vi "Move Beam.vi"(10 "Beam":refnum<class "Beam.lvclass">, 11 "Maze In":refnum<class "Maze.lvclass">) -> (2 "Beams":refnum<class "Beam.lvclass">[](array[class]), 3 "Maze Out":refnum<class "Maze.lvclass">)   [LabVIEW 2021, in "Maze.lvclass"]
uses:
  Maze.lvclass
  Beam/Beam.lvclass
  Maze.lvclass/Maze.ctl
  Beam/Beam.lvclass/Beam.ctl
  Beam/Read Row.vi
  Beam/Read Col.vi
  Beam/Read Direction.vi
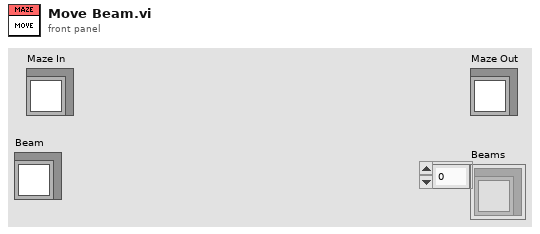
[diagram p1: front panel]
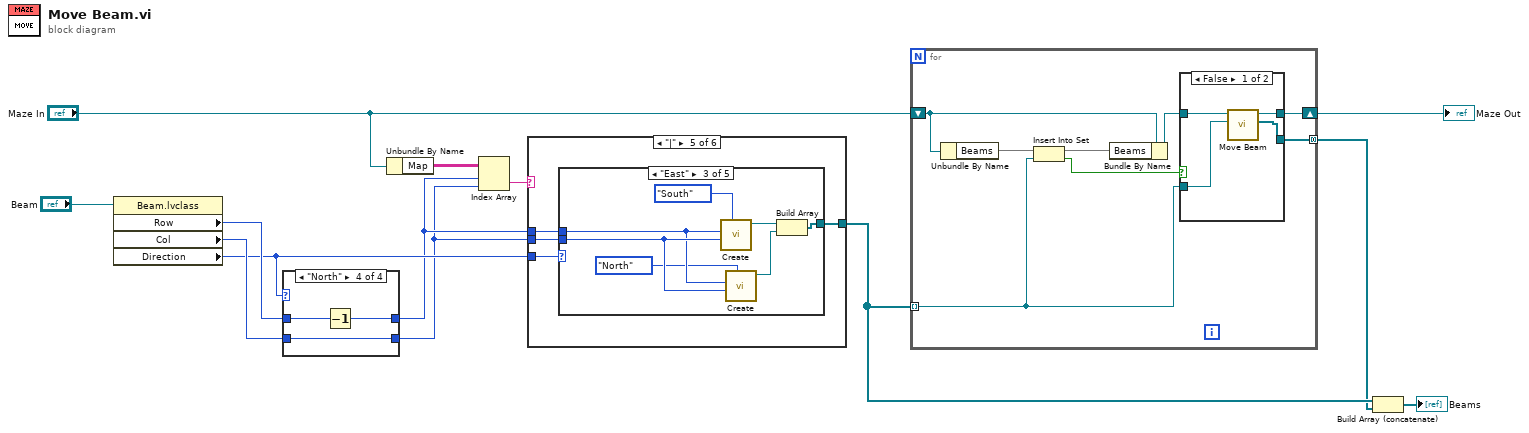
[diagram p0: block diagram]
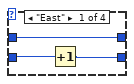
[diagram p2: hidden frame]
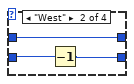
[diagram p3: hidden frame]
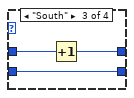
[diagram p4: hidden frame]
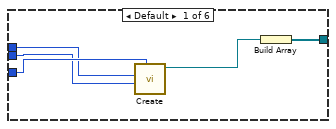
[diagram p5: hidden frame]
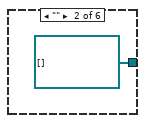
[diagram p6: hidden frame]
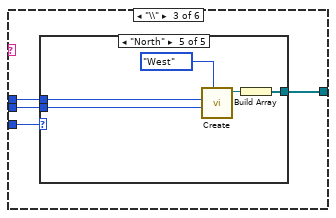
[diagram p7: hidden frame]
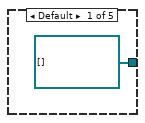
[diagram p8: hidden frame]
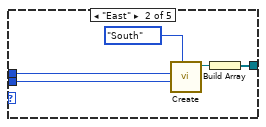
[diagram p9: hidden frame]
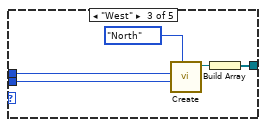
[diagram p10: hidden frame]
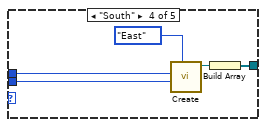
[diagram p11: hidden frame]
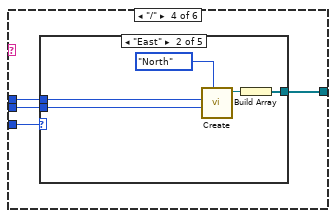
[diagram p12: hidden frame]
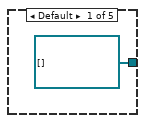
[diagram p13: hidden frame]
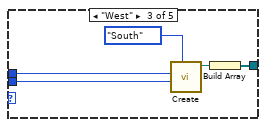
[diagram p14: hidden frame]
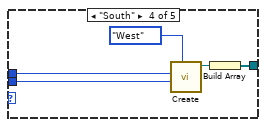
[diagram p15: hidden frame]
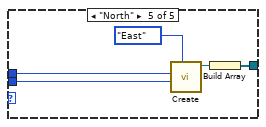
[diagram p16: hidden frame]
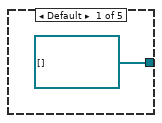
[diagram p17: hidden frame]
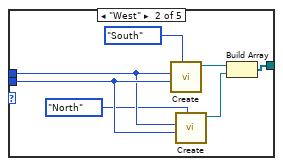
[diagram p18: hidden frame]
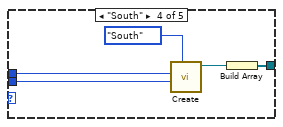
[diagram p19: hidden frame]
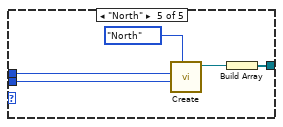
[diagram p20: hidden frame]
diagram:
  n1 = property class="Beam.lvclass"(reference="Beam") -> ("Row"=w9:i32, "Col"=w10:i32, "Direction"=w8:enum16{"North", "East", "South", "West"})  [unwired: 1 in, 2 out]
  n2 = case shown="\"North\"" w8 {
    tunnel: w10 -> [w16 w19 w22 w25]
    tunnel: w9 -> [w14 w17 w21 w24]
    tunnel: [w15 w18 w22 w25] -> w6
    tunnel: [w14 w17 w20 w23] -> w7
    frame "East" {
      n3 = Increment(x=w16) -> (x+1=w15:i32)
    }
    frame "West" {
      n4 = Decrement(x=w19) -> (x-1=w18:i32)
    }
    frame "South" {
      n5 = Increment(x=w21) -> (x+1=w20:i32)
    }
    frame "North" {
      n6 = Decrement(x=w24) -> (x-1=w23:i32)
    }
  }
  n7 = Unbundle By Name("Maze In") -> ("Map"=w12:string[][])
  n8 = Index Array(array=w12, index (row)=w7, index (col)=w6) -> (element=w11:string)
  n9 = case shown="\"|\"" w11 {
    tunnel: w8 -> [w30 _ w35 w60 w85 w114]
    tunnel: w6 -> [w28 _ w34 w59 w84 w113]
    tunnel: w7 -> [w29 _ w33 w58 w83 w112]
    tunnel: [w27 refnum<class "Beam.lvclass">[] [] w32 w57 w82 w111] -> w5
    frame Default {
      n10 = call "Create.vi"("Direction"=w30, "Col"=w28, "Row"=w29) -> ("Beam"=w26:refnum<class "Beam.lvclass">)  [unwired: 7 in, 1 out]
      n11 = Build Array(w26) -> (w27:refnum<class "Beam.lvclass">[])
    }
    frame "" {
    }
    frame "\\" {
      n12 = case shown="\"North\"" w35 {
        tunnel: w34 -> [_ w40 w45 w50 w55]
        tunnel: w33 -> [_ w39 w44 w49 w54]
        tunnel: [refnum<class "Beam.lvclass">[] [] w37 w42 w47 w52] -> w32
        frame Default {
        }
        frame "East" {
          n13 = call "Create.vi"("Direction"=enum16{"North", "East", "South", "West"}."South", "Col"=w40, "Row"=w39) -> ("Beam"=w38:refnum<class "Beam.lvclass">)  [unwired: 7 in, 1 out]
          n14 = Build Array(w38) -> (w37:refnum<class "Beam.lvclass">[])
        }
        frame "West" {
          n15 = call "Create.vi"("Direction"=enum16{"North", "East", "South", "West"}."North", "Col"=w45, "Row"=w44) -> ("Beam"=w43:refnum<class "Beam.lvclass">)  [unwired: 7 in, 1 out]
          n16 = Build Array(w43) -> (w42:refnum<class "Beam.lvclass">[])
        }
        frame "South" {
          n17 = call "Create.vi"("Direction"=enum16{"North", "East", "South", "West"}."East", "Col"=w50, "Row"=w49) -> ("Beam"=w48:refnum<class "Beam.lvclass">)  [unwired: 7 in, 1 out]
          n18 = Build Array(w48) -> (w47:refnum<class "Beam.lvclass">[])
        }
        frame "North" {
          n19 = call "Create.vi"("Direction"=enum16{"North", "East", "South", "West"}."West", "Col"=w55, "Row"=w54) -> ("Beam"=w53:refnum<class "Beam.lvclass">)  [unwired: 7 in, 1 out]
          n20 = Build Array(w53) -> (w52:refnum<class "Beam.lvclass">[])
        }
      }
    }
    frame "/" {
      n21 = case shown="\"East\"" w60 {
        tunnel: w59 -> [_ w65 w70 w75 w80]
        tunnel: w58 -> [_ w64 w69 w74 w79]
        tunnel: [refnum<class "Beam.lvclass">[] [] w62 w67 w72 w77] -> w57
        frame Default {
        }
        frame "East" {
          n22 = call "Create.vi"("Direction"=enum16{"North", "East", "South", "West"}."North", "Col"=w65, "Row"=w64) -> ("Beam"=w63:refnum<class "Beam.lvclass">)  [unwired: 7 in, 1 out]
          n23 = Build Array(w63) -> (w62:refnum<class "Beam.lvclass">[])
        }
        frame "West" {
          n24 = call "Create.vi"("Direction"=enum16{"North", "East", "South", "West"}."South", "Col"=w70, "Row"=w69) -> ("Beam"=w68:refnum<class "Beam.lvclass">)  [unwired: 7 in, 1 out]
          n25 = Build Array(w68) -> (w67:refnum<class "Beam.lvclass">[])
        }
        frame "South" {
          n26 = call "Create.vi"("Direction"=enum16{"North", "East", "South", "West"}."West", "Col"=w75, "Row"=w74) -> ("Beam"=w73:refnum<class "Beam.lvclass">)  [unwired: 7 in, 1 out]
          n27 = Build Array(w73) -> (w72:refnum<class "Beam.lvclass">[])
        }
        frame "North" {
          n28 = call "Create.vi"("Direction"=enum16{"North", "East", "South", "West"}."East", "Col"=w80, "Row"=w79) -> ("Beam"=w78:refnum<class "Beam.lvclass">)  [unwired: 7 in, 1 out]
          n29 = Build Array(w78) -> (w77:refnum<class "Beam.lvclass">[])
        }
      }
    }
    frame "|" {
      n30 = case shown="\"East\"" w85 {
        tunnel: w84 -> [_ w90 w97 w102 w107]
        tunnel: w83 -> [_ w89 w96 w101 w106]
        tunnel: [refnum<class "Beam.lvclass">[] [] w91 w98 w103 w108] -> w82
        frame Default {
        }
        frame "West" {
          n31 = call "Create.vi"("Direction"=enum16{"North", "East", "South", "West"}."South", "Col"=w90, "Row"=w89) -> ("Beam"=w92:refnum<class "Beam.lvclass">)  [unwired: 7 in, 1 out]
          n32 = call "Create.vi"("Direction"=enum16{"North", "East", "South", "West"}."North", "Col"=w90, "Row"=w89) -> ("Beam"=w87:refnum<class "Beam.lvclass">)  [unwired: 7 in, 1 out]
          n33 = Build Array(w92, w87) -> (w91:refnum<class "Beam.lvclass">[])
        }
        frame "East" {
          n34 = call "Create.vi"("Direction"=enum16{"North", "East", "South", "West"}."South", "Col"=w97, "Row"=w96) -> ("Beam"=w99:refnum<class "Beam.lvclass">)  [unwired: 7 in, 1 out]
          n35 = call "Create.vi"("Direction"=enum16{"North", "East", "South", "West"}."North", "Col"=w97, "Row"=w96) -> ("Beam"=w94:refnum<class "Beam.lvclass">)  [unwired: 7 in, 1 out]
          n36 = Build Array(w99, w94) -> (w98:refnum<class "Beam.lvclass">[])
        }
        frame "South" {
          n37 = call "Create.vi"("Direction"=enum16{"North", "East", "South", "West"}."South", "Col"=w102, "Row"=w101) -> ("Beam"=w104:refnum<class "Beam.lvclass">)  [unwired: 7 in, 1 out]
          n38 = Build Array(w104) -> (w103:refnum<class "Beam.lvclass">[])
        }
        frame "North" {
          n39 = call "Create.vi"("Direction"=enum16{"North", "East", "South", "West"}."North", "Col"=w107, "Row"=w106) -> ("Beam"=w109:refnum<class "Beam.lvclass">)  [unwired: 7 in, 1 out]
          n40 = Build Array(w109) -> (w108:refnum<class "Beam.lvclass">[])
        }
      }
    }
    frame "-" {
      n41 = case shown="\"West\"" w114 {
        tunnel: w113 -> [_ w119 w124 w129 w136]
        tunnel: w112 -> [_ w118 w123 w128 w135]
        tunnel: [refnum<class "Beam.lvclass">[] [] w120 w125 w130 w137] -> w111
        frame Default {
        }
        frame "North" {
          n42 = call "Create.vi"("Direction"=enum16{"North", "East", "South", "West"}."East", "Col"=w119, "Row"=w118) -> ("Beam"=w121:refnum<class "Beam.lvclass">)  [unwired: 7 in, 1 out]
          n43 = call "Create.vi"("Direction"=enum16{"North", "East", "South", "West"}."West", "Col"=w119, "Row"=w118) -> ("Beam"=w116:refnum<class "Beam.lvclass">)  [unwired: 7 in, 1 out]
          n44 = Build Array(w121, w116) -> (w120:refnum<class "Beam.lvclass">[])
        }
        frame "East" {
          n45 = call "Create.vi"("Direction"=enum16{"North", "East", "South", "West"}."East", "Col"=w124, "Row"=w123) -> ("Beam"=w126:refnum<class "Beam.lvclass">)  [unwired: 7 in, 1 out]
          n46 = Build Array(w126) -> (w125:refnum<class "Beam.lvclass">[])
        }
        frame "West" {
          n47 = call "Create.vi"("Direction"=enum16{"North", "East", "South", "West"}."West", "Col"=w129, "Row"=w128) -> ("Beam"=w131:refnum<class "Beam.lvclass">)  [unwired: 7 in, 1 out]
          n48 = Build Array(w131) -> (w130:refnum<class "Beam.lvclass">[])
        }
        frame "South" {
          n49 = call "Create.vi"("Direction"=enum16{"North", "East", "South", "West"}."East", "Col"=w136, "Row"=w135) -> ("Beam"=w138:refnum<class "Beam.lvclass">)  [unwired: 7 in, 1 out]
          n50 = call "Create.vi"("Direction"=enum16{"North", "East", "South", "West"}."West", "Col"=w136, "Row"=w135) -> ("Beam"=w133:refnum<class "Beam.lvclass">)  [unwired: 7 in, 1 out]
          n51 = Build Array(w138, w133) -> (w137:refnum<class "Beam.lvclass">[])
        }
      }
    }
  }
  n52 = for {
    tunnel: w5 -> [w143] mode=indexing
    shift-right: [w147] -> w4
    shift-left: "Maze In" -> [w146]
    tunnel: [w140] -> w2 mode=concatenating
    n53 = Unbundle By Name(w146) -> ("Beams"=w144:set{refnum<class "Beam.lvclass">})
    n54 = Insert Into Set(10:w143, 11:w144) -> (2:w141:bool, 3:w142:set{refnum<class "Beam.lvclass">})
    n55 = Bundle By Name(cluster=w146, "Beams"=w142) -> (w145:refnum<class "Maze.lvclass">)
    n56 = case shown="False" w141 {
      tunnel: [w151 w153] -> w147
      tunnel: w145 -> [w150 w153]
      tunnel: w143 -> [w149 _]
      tunnel: [w148 refnum<class "Beam.lvclass">[] [] ("Beams")] -> w140
      frame False {
        n57 = call "Move Beam.vi"("Beam"=w149, "Maze In"=w150) -> ("Beams"=w148:refnum<class "Beam.lvclass">[], "Maze Out"=w151:refnum<class "Maze.lvclass">)  [unwired: 8 in]
      }
      frame True {
      }
    }
  }
  "Maze Out" <- w4
  n58 = Build Array (concatenate)(w5, w2) -> (→"Beams":refnum<class "Beam.lvclass">[])
